vi "Sonuç_Led_Rengi.vi"() -> (0 "Array":cluster{u32, u32}[](array[cluster]))   [LabVIEW 2014]
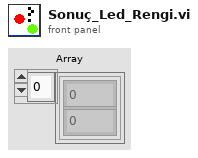
[diagram p1: front panel]
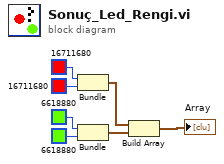
[diagram p0: block diagram]
diagram:
  n1 = Bundle(u32 16711680, u32 16711680) -> (w3:cluster{u32, u32})  [unwired: 1 in]
  n2 = Bundle(u32 6618880, u32 6618880) -> (w6:cluster{u32, u32})  [unwired: 1 in]
  n3 = Build Array(w3, w6) -> (→"Array":cluster{u32, u32}[])
